vi "RT IO Loop.vi"(7 "FPGA I/O IRQ Number(s)":i32, 8 "error in":errorcluster, 9 "response queue":refnum<queue>, 10 "message queue":refnum<queue>, 11 "FPGA VI Reference in":refnum<k20>) -> (2 "REQUEST_ID":u64)   [LabVIEW 2018]
uses:
  Message Queue/Message Cluster.ctl
  Type Def Ctrls/RT ctrls/data summary.ctl
  <vilib>/Utility/error.llb/Error Cluster From Error Code.vi
  <vilib>/rvi/errors/niLvFpgaAdjustHostInterfaceError.vi
  <vilib>/RVI Host/nirviSupport.llb/nirviErrorClusterFromErrorCode.vi
  Globals/RT AND FPGA SETTINGS.vi
  <vilib>/rvi/interface/nirviReadWriteControl/nirviReadWriteControl.xnode
  <vilib>/rvi/interface/nirviMethod/nirviMethod.xnode
  <vilib>/rvi/interface/nirviMethod/StockFPGA_InlinedMethodWaitForSingleIRQ.vi
  <vilib>/FPGAPlugInAG/Dynamic/niLvFpga_WaitOnIrq_Dynamic.vi
  <vilib>/FPGAPlugInAG/Dynamic/niLvFpga_AcknowledgeIrq_Dynamic.vi
  Message Queue/Message Queue.lvlib
  NiFpgaLv.dll
  <vilib>/rvi/interface/Simulation/niFpgaSimulationCallBeginRW.vi
  <vilib>/FPGAPlugInAG/Dynamic/niLvFpga_WriteFifo_Dynamic.vi
  <vilib>/rvi/errors/niLvFpgaMergeErrorWithErrorCode.vi
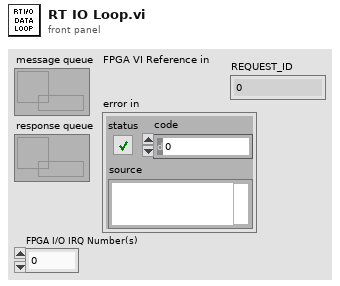
[diagram p1: front panel]
types:
  T1 = enum16{"Safe State", "I/O with PID Control", "Fast Output Only", "NOT_READY"}
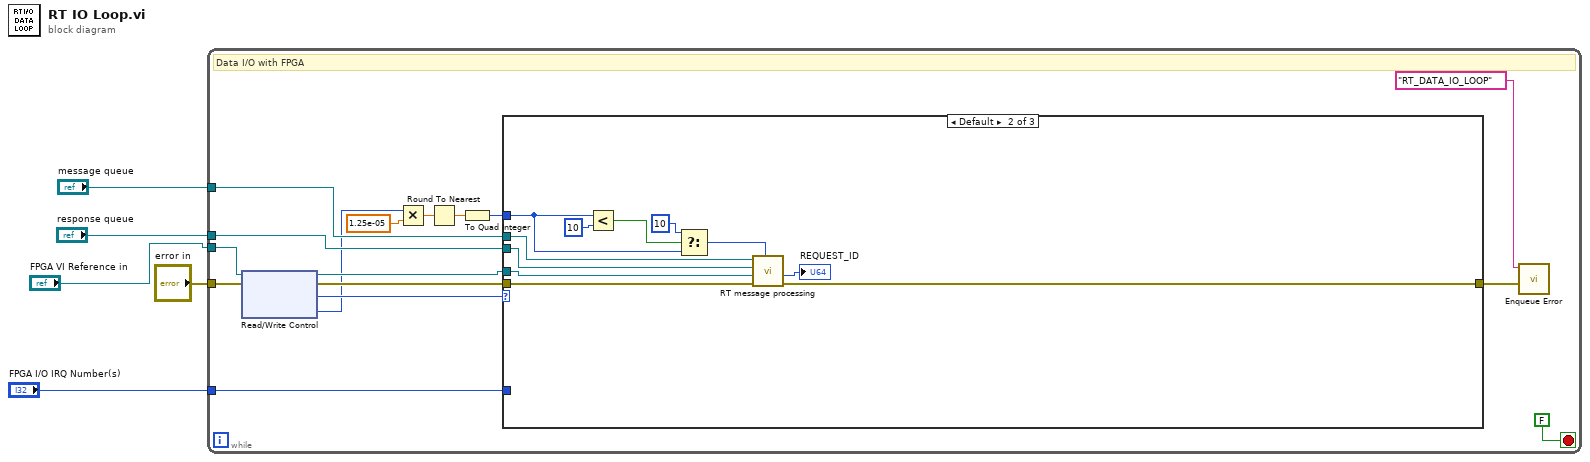
[diagram p0: block diagram]
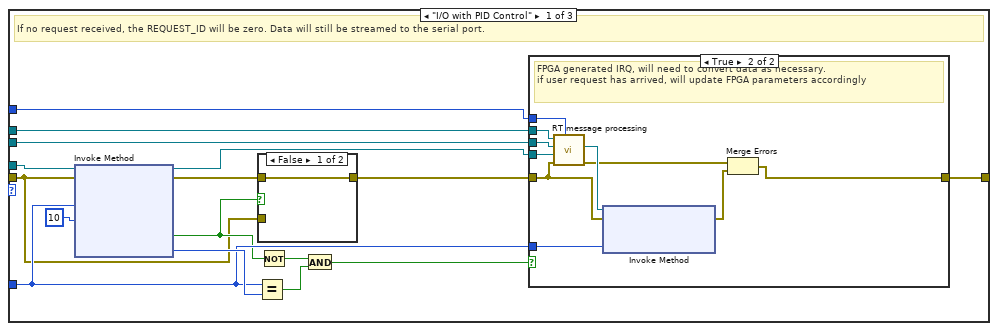
[diagram p2: hidden frame]
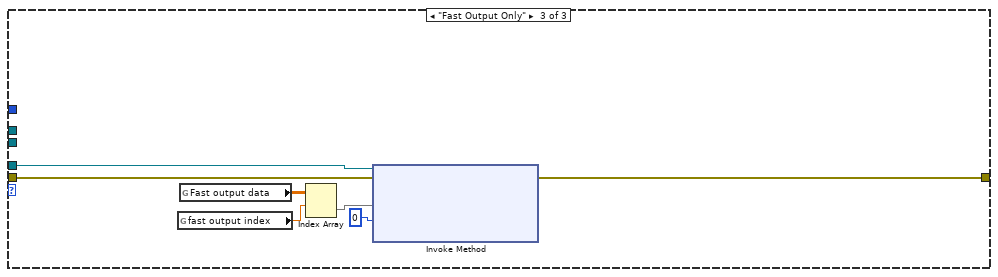
[diagram p5: hidden frame]
diagram:
  n1 = while {
    tunnel: "FPGA I/O IRQ Number(s)" -> [w21]
    tunnel: "message queue" -> [w17]
    tunnel: "error in" -> [w16]
    tunnel: "FPGA VI Reference in" -> [w20]
    tunnel: "response queue" -> [w15]
    stop <- FALSE stop-if-true
    # "Data I/O with FPGA"
    n2 = xnode "Read/Write Control"("FPGA VI Reference In"=w20, "error in"=w16) -> ("FPGA VI Reference Out"=w19:refnum<k20>, "error out"=w18:errorcluster, "FPGA state"=w12:T1, "ticks"=w11:i64)
    n3 = Multiply(x=w11, y=1.25e-05) -> (x*y=w9:dbl)
    n4 = Round To Nearest(number=w9) -> (nearest integer value=w8:dbl)
    n5 = To Quad Integer(1:w8) -> (0:w7:i64)
    n6 = case shown="Default" w12 {
      tunnel: w19 -> [w37 w59 w66]
      tunnel: w18 -> [w25 w58 w68]
      tunnel: w21 -> [w30 _ _]
      tunnel: w17 -> [w31 w61 _]
      tunnel: w15 -> [w29 w60 _]
      tunnel: [w24 w57 w67] -> w14
      tunnel: w7 -> [w22 w54 _]
      frame "I/O with PID Control" {
        # "If no request received, the REQUEST_ID will be zero. Data will still be streamed to the serial port."
        n7 = xnode "Invoke Method"("FPGA VI Reference In"=w37, "error in"=w25, "IRQ Number(s)"=w30, "Timeout (ms)"=10) -> ("FPGA VI Reference Out"=w32:refnum<k20>, "error out"=w27:errorcluster, "Timed Out"=w28:bool, "IRQ(s) Asserted"=w33:i32)
        n8 = Equal?(x=w30, y=w33) -> (x = y?=w35:bool)
        n9 = case shown="False" w28 {
          tunnel: w27 -> [w38 _]
          tunnel: [w38 w39] -> w26
          tunnel: w25 -> [_ w39]
          frame False {
          }
          frame True {
          }
        }
        n10 = Not(x=w28) -> (.not. x?=w36:bool)
        n11 = And(x=w36, y=w35) -> (x .and. y?=w34:bool)
        n12 = case shown="True" w34 {
          tunnel: [w40 w41] -> w24
          tunnel: w26 -> [w40 w44]
          tunnel: w32 -> [_ w47]
          tunnel: w31 -> [_ w49]
          tunnel: w30 -> [_ w46]
          tunnel: w29 -> [_ w50]
          tunnel: w22 -> [_ w48]
          frame False {
          }
          frame True {
            # "FPGA generated IRQ, will need to convert data as necessary.\nif user request has arrived, will update FPGA parameters accordingly"
            n13 = call "RT message processing.vi"("timeout in ms"=w48, "error in (no error)"=w44, "FPGA VI Reference in"=w47, "serial message queue"=w50, "RT message queue"=w49) -> ("error out"=w42:errorcluster, "FPGA VI Reference Out"=w45:refnum<k20>)  [unwired: 2 in, 1 out]
            n14 = xnode "Invoke Method"("FPGA VI Reference In"=w45, "error in"=w44, "IRQ Number(s)"=w46) -> ("error out"=w43:errorcluster)  [unwired: 1 out]
            n15 = Merge Errors(w42, w43) -> (w41:errorcluster)
          }
        }
      }
      frame Default {
        n16 = Less?(x=w54, y=i64 10) -> (x < y?=w56:bool)
        n17 = Select(t=i64 10, s=w56, f=w54) -> (s? t:f=w52:i64)
        n18 = call "RT message processing.vi"("timeout in ms"=w52, "error in (no error)"=w58, "FPGA VI Reference in"=w59, "serial message queue"=w60, "RT message queue"=w61) -> ("error out"=w57:errorcluster, "REQUEST_ID"=→"REQUEST_ID":u64)  [unwired: 2 in, 1 out]
      }
      frame "Fast Output Only" {
        n19 = global read "RT AND FPGA SETTINGS.vi" "fast output index"() -> (w64:dbl)
        n20 = global read "RT AND FPGA SETTINGS.vi" "Fast output data"() -> (w65:dbl[][])
        n21 = Index Array(array=w65, index (row)=w64) -> (element=w63:dbl[])  [unwired: 1 in]
        n22 = xnode "Invoke Method"("FPGA VI Reference In"=w66, "error in"=w68, "Data"=w63, "Timeout (ms)"=0) -> ("error out"=w67:errorcluster)  [unwired: 2 out]
      }
    }
    n23 = call "Enqueue Error.vi"("error to process"=w14, "Block information (which loop the error happens)"="RT_DATA_IO_LOOP") -> ()  [unwired: 9 in, 1 out]
  }
